vi "Data Parser.vi"(11 "Raw Data":fxp<+/-,22,11>[](array[numeric])) -> (0 "Data Out":dbl[][](array[numeric]), 1 "Day":i32, 2 "CSV String":string, 3 "Anomaly Array":i32[](array[numeric]))   [LabVIEW 2019]
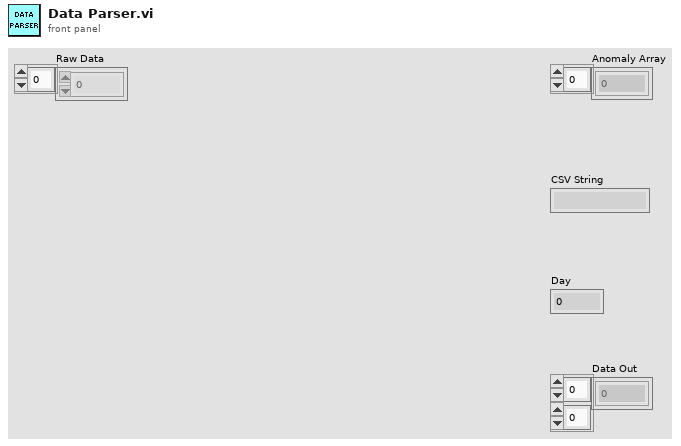
[diagram p1: front panel]
types:
  T1 = typedef "LVDateTimeRec.ctl" = cluster{"fractional second":dbl, "second":i32, "minute":i32, "hour":i32, "day of month":i32, "month":i32, "year":i32, "day of week":i32, "day of year":i32, "DST":i32}
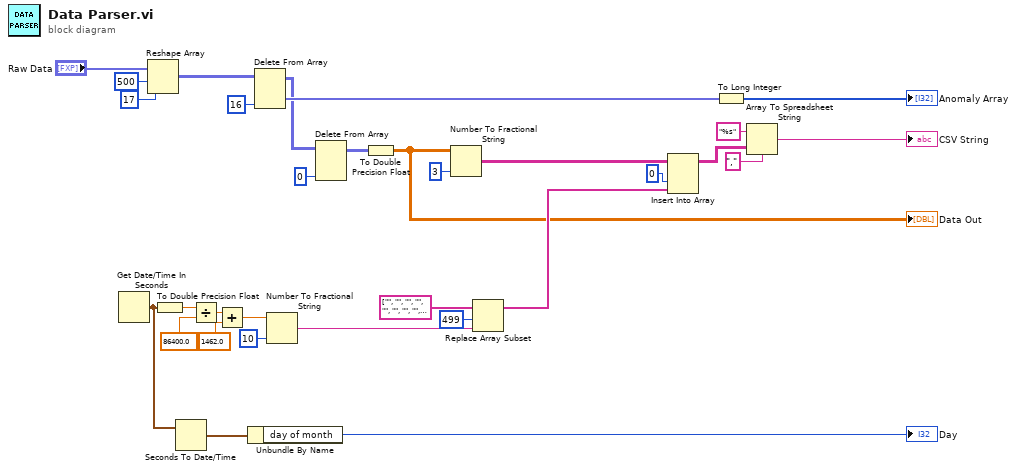
[diagram p0: block diagram]
diagram:
  n1 = Get Date/Time In Seconds() -> (seconds since 1Jan1904=w20:timestamp)
  n2 = Reshape Array("Raw Data", 500 ("dimension size"), 17 ("dimension size")) -> (w28:fxp<+/-,22,11>[][])
  n3 = To Double Precision Float(number=w20) -> (double precision float=w17:dbl)
  n4 = Seconds To Date/Time(time stamp (now)=w20) -> (date time rec=w21:T1)  [unwired: 1 in]
  n5 = Divide(x=w17, y=86400.0) -> (x/y=w15:dbl)
  n6 = Add(x=w15, y=1462.0) -> (x+y=w18:dbl)
  n7 = Unbundle By Name(w21) -> ("day of month"=→"Day":i32)
  n8 = Delete From Array(array=w28, index (col)=16 ("disabled index (col)")) -> (deleted portion=w30:fxp<+/-,22,11>[], array with subset deleted=w5:fxp<+/-,22,11>[][])  [unwired: 2 in]
  n9 = Number To Fractional String(number=w18, precision (6)=i16 10) -> (F-format string=w19:string)  [unwired: 2 in]
  n10 = Delete From Array(array=w5, index (col)=0 ("disabled index (col)")) -> (array with subset deleted=w3:fxp<+/-,22,11>[][])  [unwired: 2 in, 1 out]
  n11 = To Double Precision Float(number=w3) -> (double precision float=w2:dbl[][])
  "Data Out" <- w2
  n12 = Number To Fractional String(number=w2, precision (6)=i16 3) -> (F-format string=w12:string[][])  [unwired: 2 in]
  n13 = Replace Array Subset(array=string[] ["", "", "", "", "", "", "", "", "", "", "", "", "", "", "", "", "", "", "", "", "", "", "", "", "", "", "", "", "", "", "", "", "", "", "", "", "", "", "", "", "", "", "", "", "", "", "", "", "", "", "", "", "", "", "", "", "", "", "", "", "", "", "", "", "", "", "", "", "", "", "", "", "", "", "", "", "", "", "", "", "", "", "", "", "", "", "", "", "", "", "", "", "", "", "", "", "", "", "", "", "", "", "", "", "", "", "", "", "", "", "", "", "", "", "", "", "", "", "", "", "", "", "", "", "", "", "", "", "", "", "", "", "", "", "", "", "", "", "", "", "", "", "", "", "", "", "", "", "", "", "", "", "", "", "", "", "", "", "", "", "", "", "", "", "", "", "", "", "", "", "", "", "", "", "", "", "", "", "", "", "", "", "", "", "", "", "", "", "", "", "", "", "", "", "", "", "", "", "", "", "", "", "", "", "", "", "", "", "", "", "", "", "", "", "", "", "", "", "", "", "", "", "", "", "", "", "", "", "", "", "", "", "", "", "", "", "", "", "", "", "", "", "", "", "", "", "", "", "", "", "", "", "", "", "", "", "", "", "", "", "", "", "", "", "", "", "", "", "", "", "", "", "", "", "", "", "", "", "", "", "", "", "", "", "", "", "", "", "", "", "", "", "", "", "", "", "", "", "", "", "", "", "", "", "", "", "", "", "", "", "", "", "", "", "", "", "", "", "", "", "", "", "", "", "", "", "", "", "", "", "", "", "", "", "", "", "", "", "", "", "", "", "", "", "", "", "", "", "", "", "", "", "", "", "", "", "", "", "", "", "", "", "", "", "", "", "", "", "", "", "", "", "", "", "", "", "", "", "", "", "", "", "", "", "", "", "", "", "", "", "", "", "", "", "", "", "", "", "", "", "", "", "", "", "", "", "", "", "", "", "", "", "", "", "", "", "", "", "", "", "", "", "", "", "", "", "", "", "", "", "", "", "", "", "", "", "", "", "", "", "", "", "", "", "", "", "", "", "", "", "", "", "", "", "", "", "", "", "", "", "", "", "", "", "", "", "", "", "", "", "", "", "", "", "", "", "", "", "", "", "", "", "", "", "", "", "", "", "", "", "", "", "", "", "", "", "", "", "", ""], new element=w19, index=499) -> (w9:string[])
  n14 = Insert Into Array(array=w12, index (col)=0 ("disabled index (col)"), new element=w9) -> (w6:string[][])  [unwired: 1 in]
  n15 = To Long Integer(number=w30) -> (32bit integer=→"Anomaly Array":i32[])
  n16 = Array To Spreadsheet String(delimiter (Tab)=",", array=w6, 3:"%s" ("format string")) -> (spreadsheet string=→"CSV String":string)
